vi "Example - Cluster retrieve rulers - Copy.vi"() -> ()   [LabVIEW 2017]
uses:
  db531f95-5889-428f-99e9-9bee3c65bca8.vi
  91606217-0aa9-4d15-96b7-8b297c548ea6.vi
  1666e5c6-ebfe-49ef-8ce9-ca26aba7fc85.vi
  0581107d-8152-4841-aa39-46f148f37cd2.vi
  8f60ddcf-0cb1-4fc8-acc6-41852b9c13b8.vi
  64d8a324-6c64-445f-bd9e-bddeadd68038.vi
  2fe488ef-b7bb-44d0-a25d-5ffd90c1f184.vi
  a9cae98a-f907-4981-8728-e4dab4e61435.vi
  API-String-Arugments-Support/_Support/Data To API String Arguments.vi
  API-String-Arugments-Support/API String Arguments Support.lvlib
panel:
  out "output cluster 7":T1
  out "output cluster 6":T1
  out "output cluster 5":T1
  out "output cluster 4":T1
  out "output cluster 3":T2
  out "output cluster 2":T2
  out "output cluster 1":T2
  out "String":string
  out "data":T3
  out "error 9":errorcluster
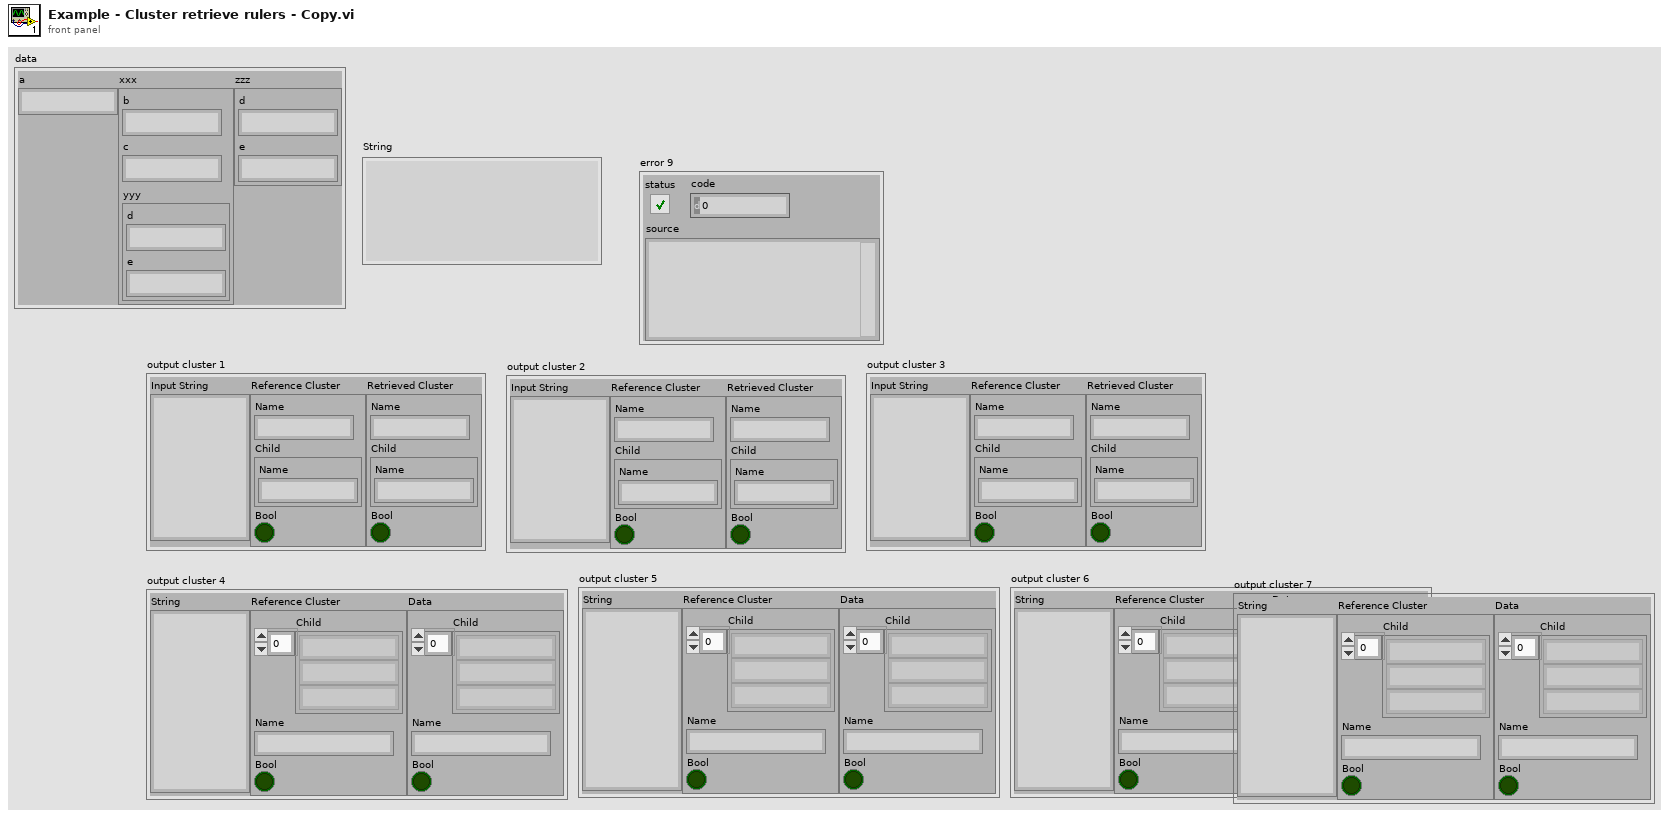
[diagram p1: front panel]
types:
  T1 = cluster{"String":string, "Reference Cluster":cluster{"Child":string[], "Name":string, "Bool":bool}, "Data":cluster{"Child":string[], "Name":string, "Bool":bool}}
  T2 = cluster{"Input String":string, "Reference Cluster":cluster{"Name":string, "Child":cluster{"Name":string}, "Bool":bool}, "Retrieved Cluster":cluster{"Name":string, "Child":cluster{"Name":string}, "Bool":bool}}
  T3 = cluster{"a":string, "xxx":cluster{"b":string, "c":string, "yyy":cluster{"d":string, "e":string}}, "zzz":cluster{"d":string, "e":string}}
  T4 = cluster{"Name":string, "Child":cluster{"Name":string}, "Bool":bool}
  T5 = cluster{"Child":string[], "Name":string, "Bool":bool}
  T6 = cluster{"String":string, "Reference Cluster":cluster{"Name":string, "Child":cluster{"Name":string}, "Bool":bool}, "Data":cluster{"Name":string, "Child":cluster{"Name":string}, "Bool":bool}}
  T7 = cluster{"String":string, "Reference Cluster 2":cluster{"Child":string[], "Name":string, "Bool":bool}, "Data":cluster{"Child":string[], "Name":string, "Bool":bool}}
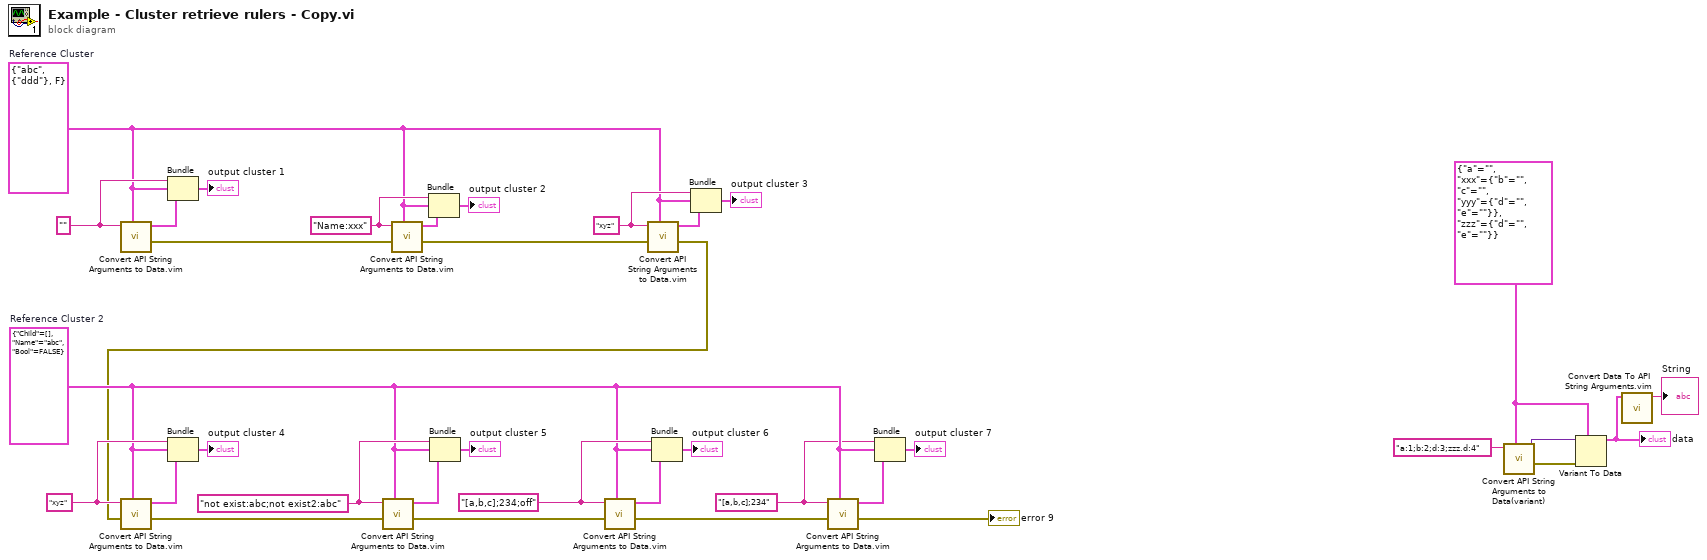
[diagram p0: block diagram]
diagram:
  w25 = "Name:xxx" ("String")
  w33 = T3 {"a"="", "xxx"={"b"="", "c"="", "yyy"={"d"="", "e"=""}}, "zzz"={"d"="", "e"=""}} ("Data 8")
  w3 = "[a,b,c];234" ("String")
  w8 = "[a,b,c];234;off" ("String")
  w12 = "not exist:abc;not exist2:abc" ("String")
  w30 = "" ("String")
  w20 = T4 {"Name"="abc", "Child"={"Name"="ddd"}, "Bool"=FALSE}  # Reference Cluster
  w18 = "xyz" ("String")
  w4 = T5 {"Child"=[], "Name"="abc", "Bool"=FALSE}  # Reference Cluster 2
  w21 = "xyz" ("String")
  n1 = call "Convert API String Arguments to Data.vim"("Type"=w20, "String"=w30) -> ("error"=w27:errorcluster, "Data"=w29:T4)  [unwired: 6 in]
  n2 = Bundle("String"=w30, "Reference Cluster"=w20, "Data"=w29) -> (→"output cluster 1":T6)  [unwired: 1 in]
  n3 = call "Convert API String Arguments to Data.vim"("Type"=w20, "error in (no error)"=w27, "String"=w25) -> ("error"=w23:errorcluster, "Data"=w24:T4)  [unwired: 5 in]
  n4 = Bundle("String"=w25, "Reference Cluster"=w20, "Data"=w24) -> (→"output cluster 2":T6)  [unwired: 1 in]
  n5 = call "Convert API String Arguments to Data.vim"("Type"=w20, "error in (no error)"=w23, "String"=w21) -> ("error"=w2:errorcluster, "Data"=w19:T4)  [unwired: 5 in]
  n6 = call "Convert API String Arguments to Data.vim"("Type"=w4, "error in (no error)"=w2, "String"=w18) -> ("error"=w13:errorcluster, "Data"=w17:T5)  [unwired: 5 in]
  n7 = Bundle("String"=w18, "Reference Cluster 2"=w4, "Data"=w17) -> (→"output cluster 4":T7)  [unwired: 1 in]
  n8 = call "Convert API String Arguments to Data.vim"("Type"=w4, "error in (no error)"=w13, "String"=w12) -> ("error"=w9:errorcluster, "Data"=w14:T5)  [unwired: 5 in]
  n9 = Bundle("String"=w12, "Reference Cluster 2"=w4, "Data"=w14) -> (→"output cluster 5":T7)  [unwired: 1 in]
  n10 = call "Convert API String Arguments to Data.vim"("Type"=w4, "error in (no error)"=w9, "String"=w8) -> ("error"=w5:errorcluster, "Data"=w11:T5)  [unwired: 5 in]
  n11 = Bundle("String"=w8, "Reference Cluster 2"=w4, "Data"=w11) -> (→"output cluster 6":T7)  [unwired: 1 in]
  n12 = Bundle("String"=w21, "Reference Cluster"=w20, "Data"=w19) -> (→"output cluster 3":T6)  [unwired: 1 in]
  n13 = call "Convert API String Arguments to Data.vim"("Type"=w4, "error in (no error)"=w5, "String"=w3) -> ("error"=→"error 9":errorcluster, "Data"=w6:T5)  [unwired: 5 in]
  n14 = Bundle("String"=w3, "Reference Cluster 2"=w4, "Data"=w6) -> (→"output cluster 7":T7)  [unwired: 1 in]
  n15 = call "Convert API String Arguments to Data(variant).vi"("Type"=w33, "String"="a:1;b:2;d:3;zzz.d:4") -> ("error"=w34:errorcluster, "Data"=w35:variant)  [unwired: 8 in]
  n16 = Variant To Data(error in=w34, type=w33, Variant=w35) -> (data=w32:T3)  [unwired: 1 out]
  "data" <- w32
  n17 = call "Convert Data To API String Arguments.vim"("data"=w32) -> ("String"=→"String":string)  [unwired: 7 in, 1 out]
